vi "读取硬件COM口.vi"(8 "error in (no error)":errorcluster caption="错误输入（无错误）", 11 "硬件输入":refnum<class "硬件.lvclass">) -> (0 "error out":errorcluster caption="错误输出", 2 "硬件COM口":refnum<visa-resource-name>, 3 "硬件输出":refnum<class "硬件.lvclass">)   [LabVIEW 2015, in "硬件.lvlib" / "硬件.lvclass"]
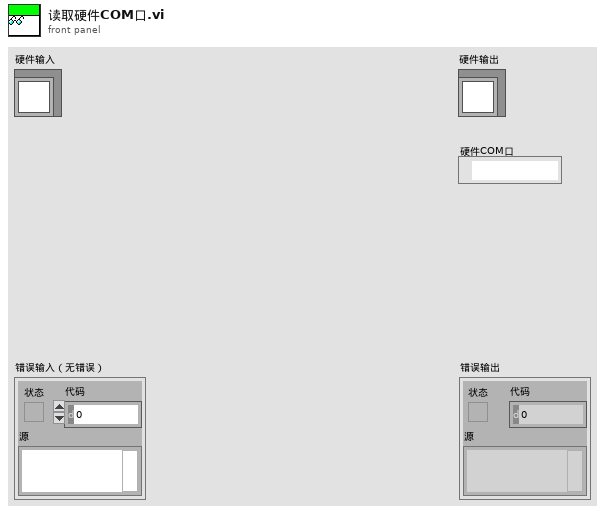
[diagram p1: front panel]
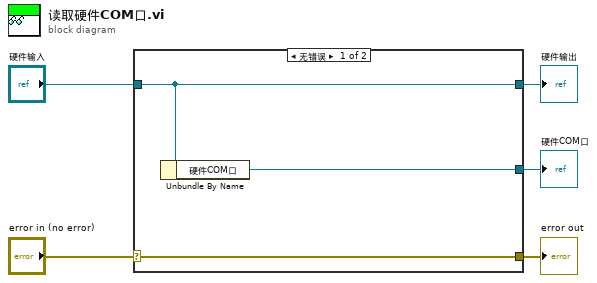
[diagram p0: block diagram]
diagram:
  n1 = case shown="无错误" "error in (no error)" {
    selector: "error in (no error)" -> [w8 w9]
    tunnel: [w8 w9] -> w4
    tunnel: [w7 w10] -> w2
    tunnel: "硬件输入" -> [w7 w10]
    tunnel: [w6 _] -> w1
    frame No Error {
      n2 = Unbundle By Name(w7) -> ("硬件COM口"=w6:refnum<visa-resource-name>)
    }
    frame Error {
    }
  }
  "error out" <- w4
  "硬件输出" <- w2
  "硬件COM口" <- w1
